vi "Publish.vi"(0 "WAMP Client in":refnum<class "WAMP Client.lvclass">, 1 "error in (no error)":errorcluster, 2 "Time out (ms)":i32=-1, 3 "Topic":string, 4 "Arguments":variant[](array[variant]), 5 "ArgumentsKw":string, 7 "Request Ack.":bool) -> (14 "WAMP Client out":refnum<class "WAMP Client.lvclass">, 15 "error out":errorcluster)   [LabVIEW 2020, in "WAMP Client.lvclass"]
uses:
  <userlib>/lvwamp/WAMP Client/WAMP Client.lvclass
  <vilib>/Utility/error.llb/Error Cluster From Error Code.vi
  <vilib>/ErrorRing/Error Ring.xnode
panel:
  out "Success?":bool
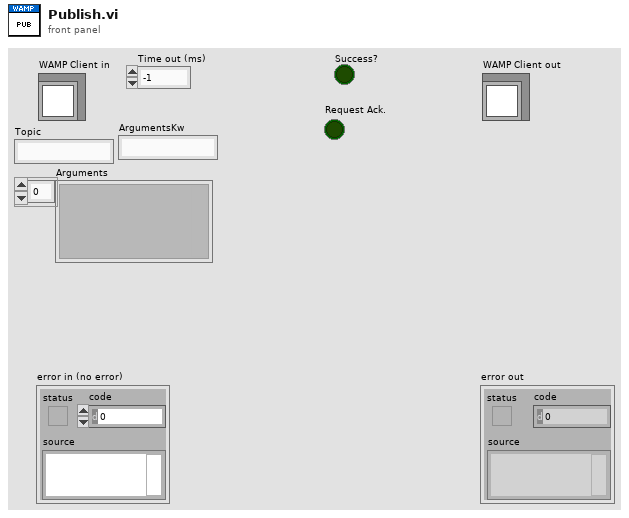
[diagram p1: front panel]
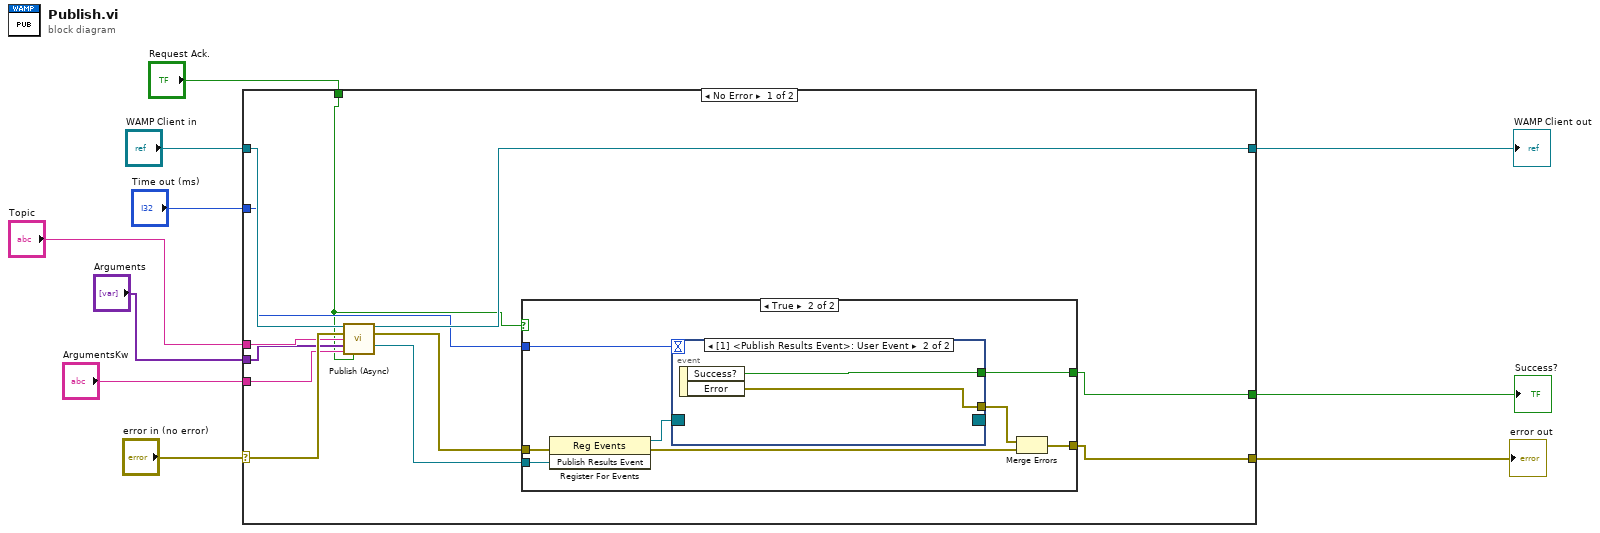
[diagram p0: block diagram]
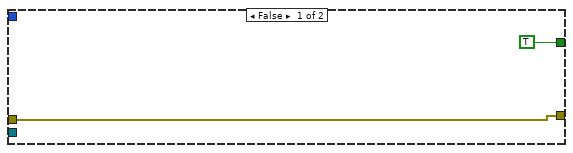
[diagram p2: hidden frame]
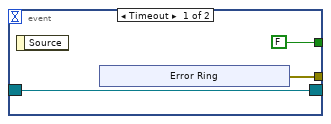
[diagram p3: hidden frame]
diagram:
  n1 = case shown="No Error" "error in (no error)" {
    selector: "error in (no error)" -> [w21 w44]
    tunnel: [w13 w44] -> w9
    tunnel: [w17 w43] -> w7
    tunnel: "WAMP Client in" -> [w22 w43]
    tunnel: "Topic" -> [w20 _]
    tunnel: "Arguments" -> [w19 _]
    tunnel: "ArgumentsKw" -> [w18 _]
    tunnel: [w14 _] -> w3
    tunnel: "Time out (ms)" -> [w12 _]
    tunnel: "Request Ack." -> [w11 _]
    frame No Error {
      n2 = call-dynamic "Publish (Async).vi"("WAMP Client in"=w22, "error in (no error)"=w21, "Topic"=w20, "Arguments"=w19, "ArgumentsKw"=w18, "Request Ack."=w11) -> ("WAMP Client out"=w17:refnum<class "WAMP Client.lvclass">, "error out"=w15:errorcluster, "Publish Results Event"=w16:refnum<user-event>)  [unwired: 7 in]
      n3 = case shown="True" w11 {
        tunnel: w16 -> [_ w32]
        tunnel: w15 -> [w23 w31]
        tunnel: [TRUE ("Success?") w29] -> w14
        tunnel: [w23 w26] -> w13
        tunnel: w12 -> [_ w25]
        frame False {
        }
        frame True {
          n4 = register-events(error in=w31, w32) -> (reference out=w30:refnum<event-registration>, error out=w28:errorcluster)  [unwired: 1 in]
          n5 = event shown="[1] <Publish Results Event>: User Event" {
            selector: w30 -> [w34 _]
            dyn-events: [w34 _] -> _
            timeout: w25 -> [_ _]
            tunnel: [FALSE ("Success?") w41] -> w29
            tunnel: [w33 w42] -> w27
            event Timeout {
              n6 = event-data() -> ()  [unwired: 1 in, 1 out]
              n7 = xnode "Error Ring"() -> ("error out"=w33:errorcluster)
            }
            event User Event {
              n8 = event-data() -> ("Success?"=w41:bool, "Error"=w42:errorcluster)  [unwired: 1 in]
            }
          }
          n9 = Merge Errors(w27, w28) -> (w26:errorcluster)
        }
      }
    }
    frame Error {
    }
  }
  "error out" <- w9
  "WAMP Client out" <- w7
  "Success?" <- w3
